vi "Y_to_S.vi"(2 "error in (no error)":errorcluster, 3 "Reference Impedance":dbl=50.0, 4 "Input Y-parameter Trace Array":T2(array[cluster]) {"Freq (Hz)" format="%.2e"; "Y-parameter Array" format="%.2f"}) -> (0 "error out":errorcluster, 1 "Output S-parameter Trace Array":T1(array[cluster]) {"Freq (Hz)" format="%.2e"; "S-parameter Array" format="%.2f"})   [LabVIEW 2017]
uses:
  <vilib>/Analysis/_algsub.llb/Complex Matrix Norm.vi
  <vilib>/Analysis/baseanly.llb/Complex A x B.vi
  <vilib>/Analysis/baseanly.llb/Complex Inverse Matrix.vi
  <vilib>/Analysis/NI_AALBase.lvlib
  <vilib>/Analysis/NI_AALPro.lvlib
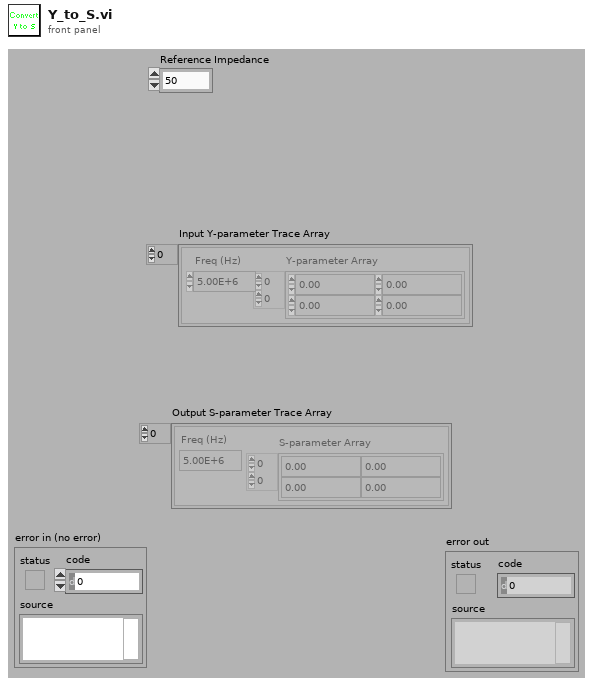
[diagram p1: front panel]
types:
  T1 = cluster{"Freq (Hz)":dbl, "S-parameter Array":csg[][]}[]
  T2 = cluster{"Freq (Hz)":dbl, "Y-parameter Array":csg[][]}[]
  T3 = typedef "NI_Matrix.lvlib/ComplexMatrix.ctl" = cdb[][]
  T4 = cluster{"Freq (Hz)":dbl, "S-parameter Array":csg[][]}
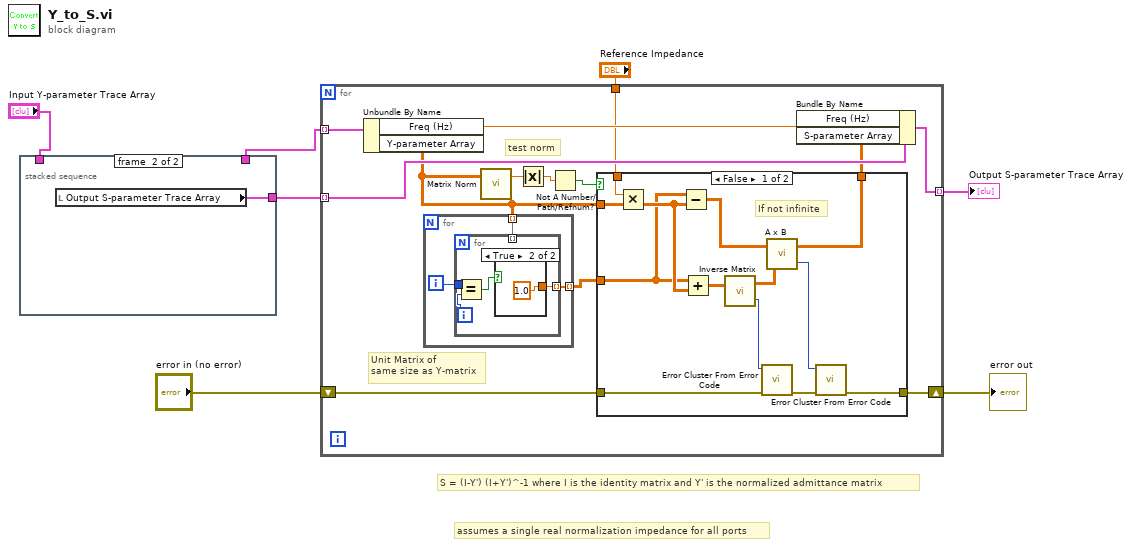
[diagram p0: block diagram]
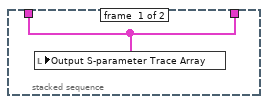
[diagram p2: hidden frame]
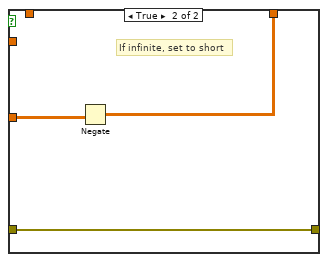
[diagram p3: hidden frame]
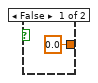
[diagram p4: hidden frame]
diagram:
  # "assumes a single real normalization impedance for all ports"
  # "S = (I-Y') (I+Y')^-1 where I is the identity matrix and Y' is the normalized admittance matrix"
  n1 = stacked-sequence {
    tunnel: "Input Y-parameter Trace Array" -> [w8 _]
    tunnel: [w8 _] -> w3
    tunnel: [_ w9] -> w2
    frame #0 {
      n2 = local write "Output S-parameter Trace Array"(w8) -> ()
    }
    frame #1 {
      n3 = local read "Output S-parameter Trace Array"() -> (w9:T1)
    }
  }
  n4 = for {
    tunnel: w3 -> [w22] mode=indexing
    tunnel: [w20] -> w7 mode=indexing
    shift-right: [w18] -> w5
    shift-left: "error in (no error)" -> [w19]
    tunnel: w2 -> [w17] mode=indexing
    tunnel: "Reference Impedance" -> [w16]
    # "test norm"
    # "Unit Matrix of\nsame size as Y-matrix"
    n5 = Unbundle By Name(w22) -> ("Freq (Hz)"=w21:dbl, "Y-parameter Array"=w15:csg[][])
    n6 = for {
      tunnel: w15 -> [w41] mode=indexing
      tunnel: [w39] -> w13 mode=indexing
      i -> [w40]
      n7 = for {
        tunnel: w41 -> [_] mode=indexing
        tunnel: w40 -> [w44]
        tunnel: [w42] -> w39 mode=indexing
        i -> [w45]
        n8 = Equal?(x=w44, y=w45) -> (x = y?=w43:bool)
        n9 = case shown="True" w43 {
          tunnel: [0.0 1.0] -> w42
          frame False {
          }
          frame True {
          }
        }
      }
    }
    n10 = call-poly <vilib>:"Matrix Norm.vi"("Input Matrix"=w15) -> ("norm"=w14:dbl)  [unwired: 1 in, 1 out]
    n11 = Absolute Value(x=w14) -> (abs(x)=w11:dbl)
    n12 = Not A Number/Path/Refnum?(number/path/refnum=w11) -> (NaN/Path/Refnum?=w10:bool)
    n13 = case shown="False" w10 {
      tunnel: w19 -> [w30 w38]
      tunnel: [w28 w38] -> w18
      tunnel: w16 -> [w27 _]
      tunnel: w15 -> [w25 _]
      tunnel: w13 -> [w24 w37]
      tunnel: [w23 w36] -> w12
      frame False {
        # "If not infinite"
        n14 = Multiply(x=w27, y=w25) -> (x*y=w26:cdb[][])
        n15 = Subtract(x=w24, y=w26) -> (x-y=w34:cdb[][])
        n16 = Add(x=w24, y=w26) -> (x+y=w35:cdb[][])
        n17 = call-poly <vilib>:"Inverse Matrix.vi"("Input Matrix"=w35) -> ("error"=w32:i32, "Inverse Matrix"=w33:T3)  [unwired: 1 in]
        n18 = call <vilib>:"Error Cluster From Error Code.vi"("error in (no error)"=w30, "error code (0)"=w32) -> ("error out"=w29:errorcluster)  [unwired: 1 in, 6 out]
        n19 = call-poly <vilib>:"A x B.vi"("B"=w33, "A"=w34) -> ("error"=w31:i32, "A x B"=w23:T3)
        n20 = call <vilib>:"Error Cluster From Error Code.vi"("error in (no error)"=w29, "error code (0)"=w31) -> ("error out"=w28:errorcluster)  [unwired: 1 in, 6 out]
      }
      frame True {
        # "If infinite, set to short"
        n21 = Negate(x=w37) -> (-x=w36:dbl[][])
      }
    }
    n22 = Bundle By Name(cluster=w17, "Freq (Hz)"=w21, "S-parameter Array"=w12) -> (w20:T4)
  }
  "Output S-parameter Trace Array" <- w7
  "error out" <- w5
